vi "SB_fillState_run.vi"(8 "error in (no error)":errorcluster, 11 "Initial Settings":T1={"Water density"=1000.0, "SB_parameters"={"x0"=0.0, "U_full"=0.695, "U_empty"=3.67}}) -> (0 "error out":errorcluster)   [LabVIEW 2013]
uses:
  My Computer/Controls/Sensors State.ctl
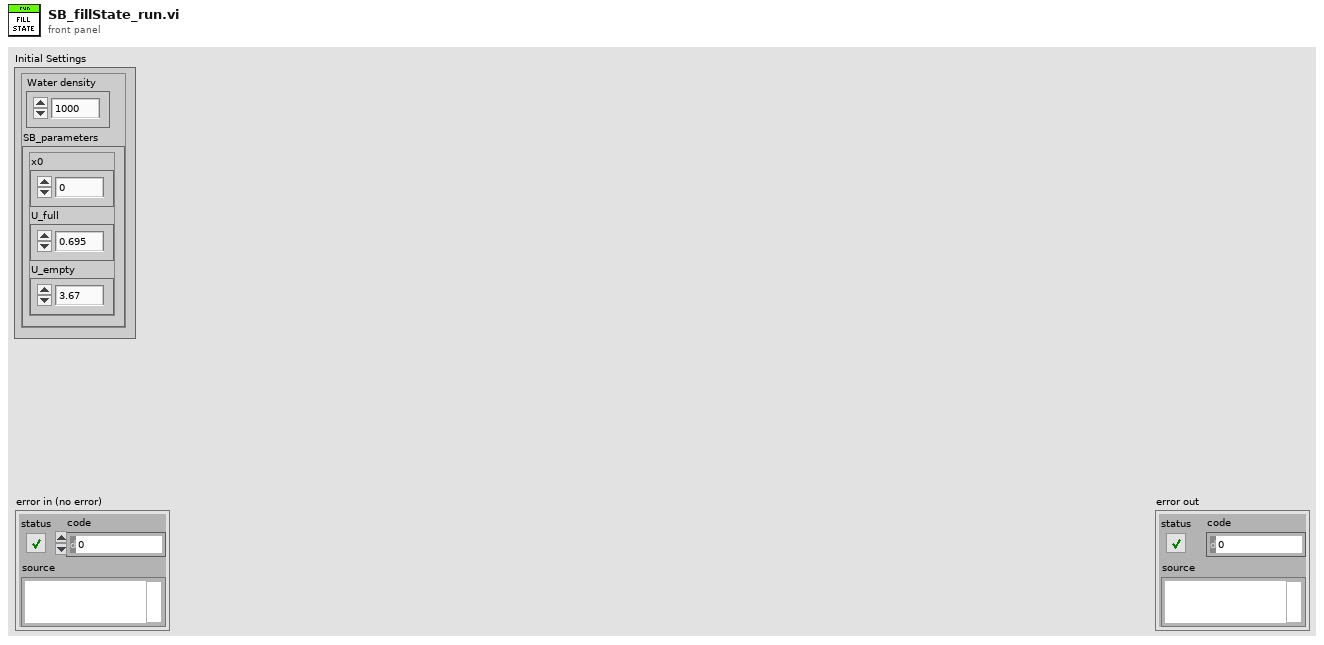
[diagram p1: front panel]
types:
  T1 = cluster{"Water density":dbl, "SB_parameters":cluster{"x0":dbl, "U_full":dbl, "U_empty":dbl}}
  T2 = typedef "Sensors State.ctl" = cluster{"Leakage-Sensor_enabled":bool, "IMU_enabled":bool, "Swimbladder Fill-State-Sensor_enabled":bool, "Flow-Sensor_enabled":bool, "Depth-Sensor_enabled":bool, "Current-Sensor_enabled":bool, "Calibrate Depth":bool, "SB_Piston_Stuck_Detect_enabled":bool, "Check_too_Deep_enabled":bool}
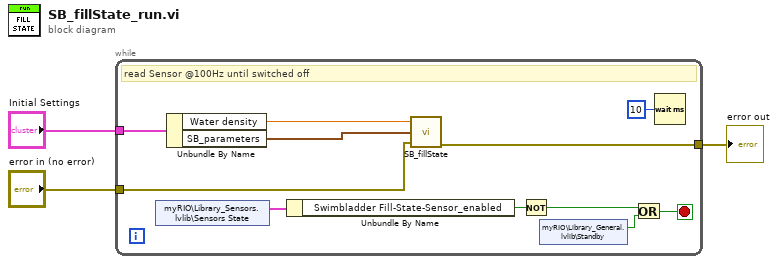
[diagram p0: block diagram]
diagram:
  n1 = while {
    tunnel: "error in (no error)" -> [w7]
    tunnel: "Initial Settings" -> [w10]
    tunnel: [w6] -> w3
    stop <- w11 stop-if-true
    # "read Sensor @100Hz until switched off"
    n2 = shared-variable "myRIO\\Library_Sensors.lvlib\\Sensors State"() -> (w5:T2)  [unwired: 1 in, 1 out]
    n3 = Unbundle By Name(w10) -> ("Water density"=w9:dbl, "SB_parameters"=w8:cluster{"x0":dbl, "U_full":dbl, "U_empty":dbl})
    n4 = Unbundle By Name(w5) -> ("Swimbladder Fill-State-Sensor_enabled"=w4:bool)
    n5 = call "SB_fillState.vi"("Water_density [kg/m^3]"=w9, "SB_parameters"=w8, "error in (no error)"=w7) -> ("error out"=w6:errorcluster)  [unwired: 4 out]
    n6 = Not(x=w4) -> (.not. x?=w12:bool)
    n7 = shared-variable "myRIO\\Library_General.lvlib\\Standby"() -> (w13:bool)  [unwired: 1 in, 1 out]
    n8 = Or(x=w12, y=w13) -> (x .or. y?=w11:bool)
    n9 = Wait (ms)(milliseconds to wait=u32 10) -> ()  [unwired: 1 out]
  }
  "error out" <- w3
